vi "3458A Cleanup Digitizing Process.vi"(8 "error in":errorcluster, 11 "session in":T1 {"channels"."Range [Vpk]" min=0.0}) -> (0 "error out":errorcluster, 3 "session out":T1 {"channels"."Range [Vpk]" min=0.0})   [LabVIEW 2013, in "3458A Virtual Digitizer.lvlib"]
doc: "Call this to cleanup whatever remained after digitizing processes. It tries to close or kill digitizing process instances for all channels, it destroys stop noifier and data queues. Call this after each digitizing process. It ignores input error."
uses:
  3458A Virtual Digitizer.lvlib
  3458A Digitizer Session.ctl
  3458A Virtual Channel Config.ctl
  Counter/Counter Session.ctl
  Counter/Counter Type.ctl
  AWG/AWG Session.ctl
  AWG/AWG Type.ctl
  3458A Sync Mode.ctl
  3458A Idn Mode.ctl
  3458A Digitizing Low Levels/Configure/Sampling Mode.ctl
  3458A Digitizing Process Options.ctl
  3458A Data Packet.ctl
  3458A Aux Record Data.ctl
  3458A Digitizing Low Levels/Configure/Level Setup.ctl
  3458A Digitizing Low Levels/Configure/First Sample Trigger.ctl
  3458A Aperture Selection Mode.ctl
  AWG/AWG.lvlib
  Counter/Counter.lvlib
  3458A Digitizing Low Levels/3458A Digitizing Low Levels.lvlib
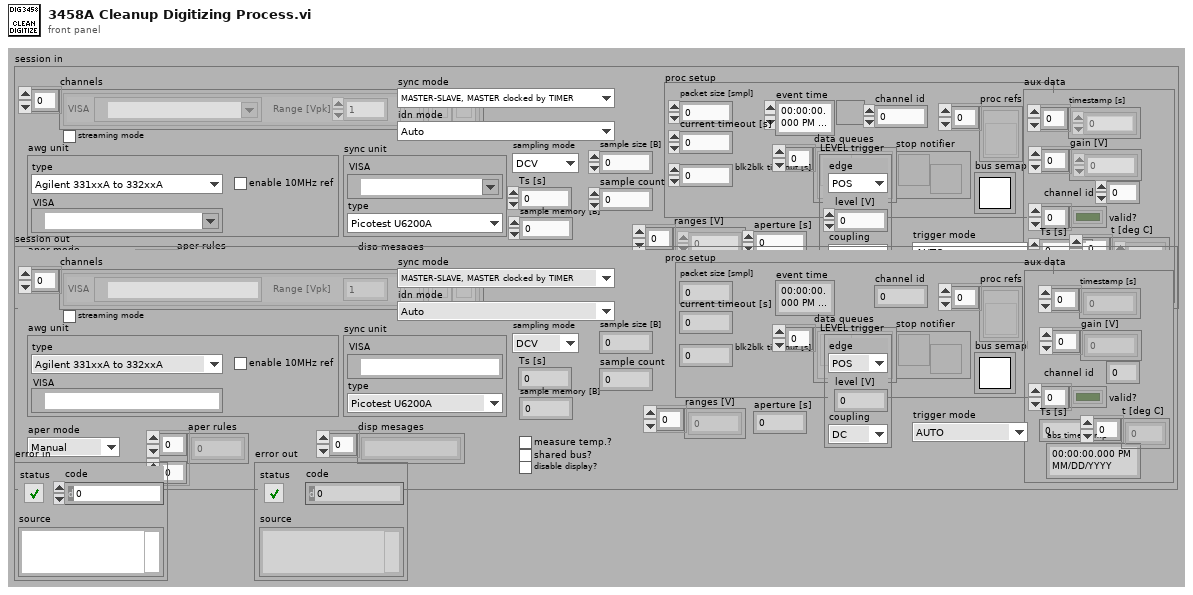
[diagram p1: front panel]
types:
  T1 = typedef "3458A Virtual Digitizer.lvlib/3458A Digitizer Session.ctl" = cluster{"channels":T2[], "sync unit":T3, "awg unit":T5, "sync mode":T7, "streaming mode":bool, "idn mode":T8, "sampling mode":T9, "Ts [s]":dbl, "sample memory [B]":i32, "proc setup":T10, "sample size [B]":i32, "sample count":i32, "aux data":T12, "ranges [V]":dbl[], "aperture [s]":dbl, "LEVEL trigger":T13, "trigger mode":T14, "measure temp.?":bool, "disp mesages":string[], "shared bus?":bool, "disable display?":bool, "aper mode":T15, "aper rules":dbl[][]}
  T2 = typedef "3458A Virtual Digitizer.lvlib/3458A Virtual Channel Config.ctl" = cluster{"VISA":refnum<visa-resource-name>, "Range [Vpk]":dbl, "btn clr":bool, "btn up":bool, "btn down":bool}
  T3 = typedef "Counter.lvlib/Counter Session.ctl" = cluster{"VISA":refnum<visa-resource-name>, "type":T4}
  T4 = typedef "Counter.lvlib/Counter Type.ctl" = enum16{"Picotest U6200A", "dummy"}
  T5 = typedef "AWG.lvlib/AWG Session.ctl" = cluster{"type":T6, "VISA":refnum<visa-resource-name>, "enable 10MHz ref":bool}
  T6 = typedef "AWG.lvlib/AWG Type.ctl" = enum16{"Agilent 331xxA to 332xxA", "Agilent 335xxA to 336xxA", "Tektronix AFG3101C", "dummy"}
  T7 = typedef "3458A Virtual Digitizer.lvlib/3458A Sync Mode.ctl" = enum16{"MASTER-SLAVE, MASTER clocked by TIMER", "MASTER-SLAVE, MASTER clocked by AWG", "ALL clocked by AWG", "MASTER-SLAVE, ALL clocked by TIMER", "ALL clocked by AWG with DFLL"}
  T8 = typedef "3458A Virtual Digitizer.lvlib/3458A Idn Mode.ctl" = enum16{"Auto", "Sequential (chn A, chn B, ...)", "From calibration string"}
  T9 = typedef "3458A Virtual Digitizer.lvlib/3458A Digitizing Low Levels.lvlib/Sampling Mode.ctl" = enum16{"DCV", "DSDC", "DSAC"}
  T10 = typedef "3458A Virtual Digitizer.lvlib/3458A Digitizing Process Options.ctl" = cluster{"channel id":i32, "packet size [smpl]":i32, "current timeout [s]":dbl, "blk2blk timeout [s]":dbl, "event time":timestamp, "stop notifier":refnum<notifier>, "data queues":refnum<queue>[], "proc refs":refnum<vi>[], "bus semaphore":T11}
  T11 = typedef "Semaphore RefNum" = refnum<k1>
  T12 = typedef "3458A Virtual Digitizer.lvlib/3458A Aux Record Data.ctl" = cluster{"channel id":i32, "valid?":bool[], "gain [V]":dbl[], "timestamp [s]":dbl[], "Ts [s]":dbl, "abs timestamp":timestamp, "t [deg C]":dbl[]}
  T13 = typedef "3458A Virtual Digitizer.lvlib/3458A Digitizing Low Levels.lvlib/Level Setup.ctl" = cluster{"edge":enum16{"POS", "NEG"}, "level [V]":dbl, "coupling":enum16{"DC", "AC"}}
  T14 = typedef "3458A Virtual Digitizer.lvlib/3458A Digitizing Low Levels.lvlib/First Sample Trigger.ctl" = enum16{"AUTO", "EXT", "SYN", "SGL", "HOLD", "LEVEL"}
  T15 = typedef "3458A Virtual Digitizer.lvlib/3458A Aperture Selection Mode.ctl" = enum16{"Manual", "Maximum", "Table"}
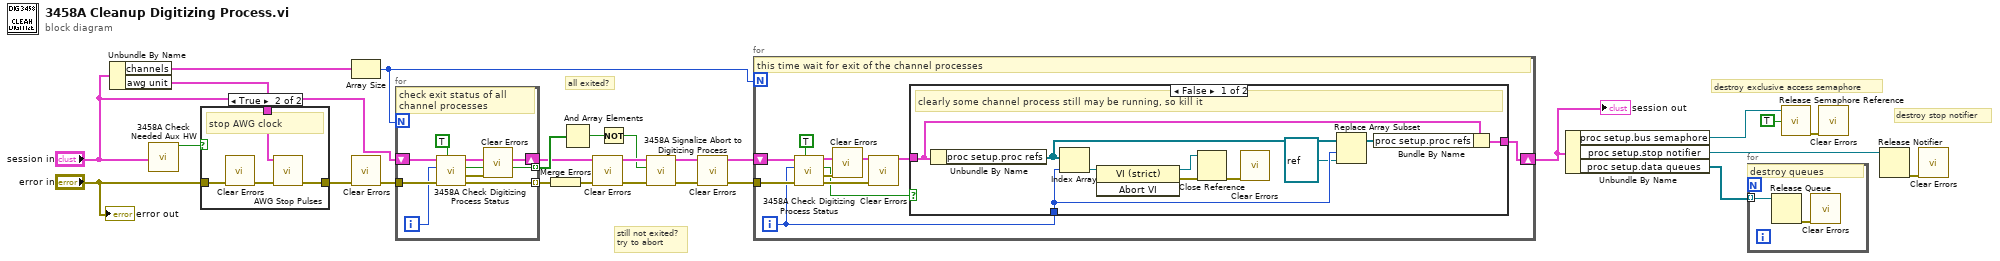
[diagram p0: block diagram]
diagram:
  # "destroy exclusive access semaphore"
  # "destroy stop notifier"
  # "still not exited?\ntry to abort"
  # "all exited?"
  n1 = Unbundle By Name("session in") -> ("channels"=w5:T2[], "awg unit"=w6:T5)
  n2 = call "3458A Check Needed Aux HW.vi"("digitizer session"="session in") -> ("uses AWG clocking?"=w7:bool)  [unwired: 13 in, 5 out]
  n3 = case shown="True" w7 {
    tunnel: [w26 w30] -> w9
    tunnel: "error in" -> [w26 w28]
    tunnel: w6 -> [_ w29]
    frame False {
    }
    frame True {
      # "stop AWG clock"
      n4 = call <vilib>:"Clear Errors.vi"("error in (no error)"=w28) -> ("error out"=w27:errorcluster)  [unwired: 6 in]
      n5 = call "AWG Stop Pulses.vi"("error in (no error)"=w27, "awg session in"=w29) -> ("error out"=w30:errorcluster)  [unwired: 8 in, 1 out]
    }
  }
  n6 = Array Size(array=w5) -> (size(s)=w14:i32)
  n7 = call <vilib>:"Clear Errors.vi"("error in (no error)"=w9) -> ("error out"=w24:errorcluster)  [unwired: 6 in]
  n8 = for {
    N: w14 -> [_]
    tunnel: [w35] -> w25 mode=indexing
    tunnel: w24 -> [w38]
    tunnel: [w32] -> w23 mode=indexing
    shift-right: [w33] -> w20
    shift-left: "session in" -> [w37]
    i -> [w36]
    # "check exit status of all\nchannel processes"
    n9 = call "3458A Check Digitizing Process Status.vi"("wait for exit (False)"=TRUE, "error in"=w38, "channel id"=w36, "digitizer session in"=w37) -> ("error out"=w32:errorcluster, "proc error out"=w34:errorcluster, "process exited?"=w35:bool, "digitizer session out"=w33:T1)  [unwired: 2 in, 2 out]
    n10 = call <vilib>:"Clear Errors.vi"("error in (no error)"=w34) -> ()  [unwired: 6 in, 1 out]
  }
  n11 = Merge Errors(w23) -> (w22:errorcluster)
  n12 = And Array Elements(Boolean array=w25) -> (logical AND=w19:bool)
  n13 = call <vilib>:"Clear Errors.vi"("error in (no error)"=w22) -> ("error out"=w21:errorcluster)  [unwired: 6 in]
  n14 = Not(x=w19) -> (.not. x?=w18:bool)
  n15 = call "3458A Signalize Abort to Digitizing Process.vi"("error in"=w21, "send abort signal? (True)"=w18, "session in"=w20) -> ("error out (copy)"=w17:errorcluster, "session out"=w15:T1)  [unwired: 7 in]
  n16 = call <vilib>:"Clear Errors.vi"("error in (no error)"=w17) -> ("error out"=w16:errorcluster)  [unwired: 6 in]
  n17 = for {
    N: w14 -> [_]
    tunnel: w16 -> [w47]
    shift-right: [w39] -> w13
    shift-left: w15 -> [w46]
    i -> [w42]
    # "this time wait for exit of the channel processes"
    n18 = call "3458A Check Digitizing Process Status.vi"("wait for exit (False)"=TRUE, "error in"=w47, "channel id"=w42, "digitizer session in"=w46) -> ("error out"=w41:errorcluster, "proc error out"=w45:errorcluster, "process exited?"=w40:bool, "digitizer session out"=w43:T1)  [unwired: 2 in, 2 out]
    n19 = call <vilib>:"Clear Errors.vi"("error in (no error)"=w45) -> ()  [unwired: 6 in, 1 out]
    n20 = call <vilib>:"Clear Errors.vi"("error in (no error)"=w41) -> ()  [unwired: 6 in, 1 out]
    n21 = case shown="False" w40 {
      tunnel: w43 -> [w50 w58]
      tunnel: w42 -> [w52 _]
      tunnel: [w48 w58] -> w39
      frame False {
        # "clearly some channel process still may be running, so kill it"
        n22 = Unbundle By Name(w50) -> ("proc setup.proc refs"=w53:refnum<vi>[])
        n23 = Index Array(array=w53, index=w52) -> (element=w57:refnum<vi>)
        n24 = invoke class="VI (strict)" method="Abort VI"(reference=w57) -> (reference out=w55:refnum<vi>, error out=w56:errorcluster)  [unwired: 2 in, 1 out]
        n25 = Close Reference(reference=w55, error in (no error)=w56) -> (error out=w54:errorcluster)
        n26 = call <vilib>:"Clear Errors.vi"("error in (no error)"=w54) -> ()  [unwired: 6 in, 1 out]
        n27 = Replace Array Subset(array=w53, new element=refnum<vi> refnum ("new element/subarray"), index=w52) -> (w49:refnum<vi>[])
        n28 = Bundle By Name(cluster=w50, "proc setup.proc refs"=w49) -> (w48:T1)
      }
      frame True {
      }
    }
  }
  "session out" <- w13
  n29 = Unbundle By Name(w13) -> ("proc setup.bus semaphore"=w2:T11, "proc setup.stop notifier"=w11:refnum<notifier>, "proc setup.data queues"=w12:refnum<queue>[])
  n30 = for {
    tunnel: w12 -> [w60] mode=indexing
    # "destroy queues"
    n31 = Release Queue(queue=w60) -> (error out=w59:errorcluster)  [unwired: 2 in, 2 out]
    n32 = call <vilib>:"Clear Errors.vi"("error in (no error)"=w59) -> ()  [unwired: 6 in, 1 out]
  }
  n33 = call <vilib>:"Release Semaphore Reference.vi"("force destroy? (F)"=TRUE, "semaphore"=w2) -> ("error out"=w1:errorcluster)  [unwired: 8 in, 1 out]
  n34 = call <vilib>:"Clear Errors.vi"("error in (no error)"=w1) -> ()  [unwired: 6 in, 1 out]
  n35 = Release Notifier(notifier=w11) -> (error out=w10:errorcluster)  [unwired: 2 in, 2 out]
  n36 = call <vilib>:"Clear Errors.vi"("error in (no error)"=w10) -> ()  [unwired: 6 in, 1 out]
  "error out" <- "error in"
